vi "Str+Unflatten.vi"(8 "error in":errorcluster, 9 "JSON Str":string, 10 "Type and Defs":variant, 11 "JSON in":refnum<class "JSON.lvclass">) -> (0 "error out":errorcluster, 2 "Data":variant, 3 "JSON out":refnum<class "JSON.lvclass">)   [LabVIEW 2017, in "Report_lib.lvlib" / "JSON.lvclass"]
doc: "This method combines and calls \ntwo methods for write JSON string\nand convert it to Data"
uses:
  JSON.lvclass
  JSON.lvclass/JSON.ctl
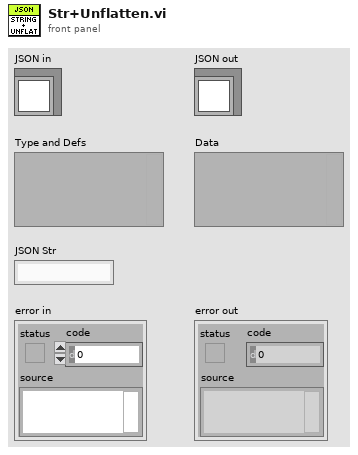
[diagram p1: front panel]
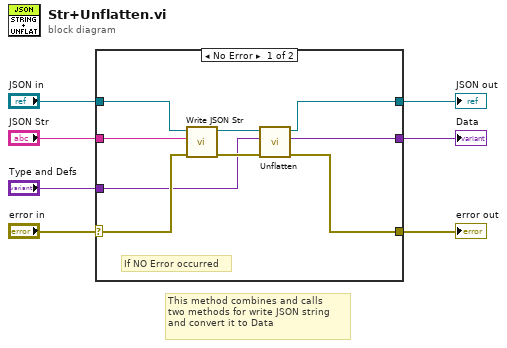
[diagram p0: block diagram]
diagram:
  # "This method combines and calls \ntwo methods for write JSON string\nand convert it to Data"
  n1 = case shown="No Error" "error in" {
    selector: "error in" -> [w13 w19]
    tunnel: [w11 w19] -> w6
    tunnel: [w14 w18] -> w4
    tunnel: "JSON in" -> [w16 w18]
    tunnel: "JSON Str" -> [w10 _]
    tunnel: "Type and Defs" -> [w9 w17]
    tunnel: [w8 w17] -> w1
    frame No Error {
      # "If NO Error occurred"
      n2 = call "Write JSON Str.vi"("error in (no error)"=w13, "JSON Str"=w10, "JSON in"=w16) -> ("error out"=w12:errorcluster, "JSON out"=w15:refnum<class "JSON.lvclass">)  [unwired: 7 in]
      n3 = call "Unflatten.vi"("error in"=w12, "Type and Defs"=w9, "JSON in"=w15) -> ("error out"=w11:errorcluster, "Data"=w8:variant, "JSON out"=w14:refnum<class "JSON.lvclass">)  [unwired: 6 in]
    }
    frame Error {
    }
  }
  "error out" <- w6
  "JSON out" <- w4
  "Data" <- w1
